vi "HTTP PUT.vi"(8 "error in (no error)":errorcluster, 9 "data":string, 10 "Endpoint":string, 11 "REST_Client in":refnum<class "REST_Client.lvclass">) -> (0 "error out":errorcluster, 1 "body":string, 2 "headers":string, 3 "REST_Client out":refnum<class "REST_Client.lvclass">)   [LabVIEW 2020, in "REST_Client.lvclass"]
uses:
  REST_Client.lvclass
  REST_Client.lvclass/REST_Client.ctl
  <vilib>/httpClient/PUTBuffer.vi
  <vilib>/httpClient/LabVIEWHTTPClient.lvlib
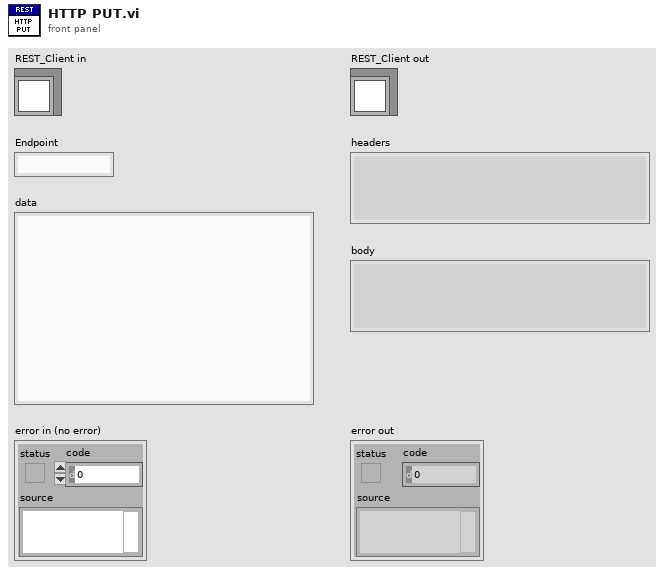
[diagram p1: front panel]
types:
  T1 = typedef "LabVIEWHTTPClient.lvlib/ClientHandle.ctl" = refnum<k1>
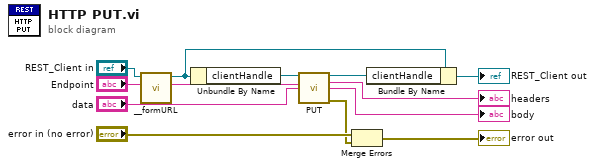
[diagram p0: block diagram]
diagram:
  n1 = call "__formURL.vi"("endPoint"="Endpoint", "REST_Client in"="REST_Client in") -> ("URL"=w11:string, "REST_Client out"=w8:refnum<class "REST_Client.lvclass">)  [unwired: 8 in]
  n2 = Unbundle By Name(w8) -> ("clientHandle"=w12:T1)
  n3 = call-poly <vilib>:"PUT.vi"("client handle"=w12, "url"=w11, "buffer"="data") -> ("client handle out"=w7:T1, "headers"=→"headers":string, "body"=→"body":string, "error out"=w2:errorcluster)  [unwired: 9 in]
  n4 = Merge Errors("error in (no error)", w2) -> (→"error out":errorcluster)
  n5 = Bundle By Name(cluster=w8, "clientHandle"=w7) -> (→"REST_Client out":refnum<class "REST_Client.lvclass">)
